vi "Inference(Image)(Batch)(Benchmark).vi"(0 "NNFE PatchCore Paths":T1={"CFG"=path "D:/Ngene/Projects_SVN/DeepLTK/R_and_D/2024_02_01_Patchcore/LabVIEW/NN_Models/PCore_L2L3_Concat_224x224/wrn/wrn_net_cfg_24_08_02__10_26_58.cfg", "BIN"=path "D:/Ngene/Projects_SVN/DeepLTK/R_and_D/2024_02_01_Patchcore/LabVIEW/NN_Models/PCore_L2L3_Concat_224x224/wrn/wrn_weights_24_08_02__10_26_58.bin"}, 1 "NNPC_Setup":T2={"Input_Dims"={"C"=3, "H"=224, "W"=224}, "mBatch"=8, "Device"=enum."GPU", "GPU Id"=0}, 2 "Feature_Scorer_Params":T5={"Nearest_Neighbors"=1, "Calculate Anomaly Map"=TRUE, "Gaussian_Blur"={"Kernel_Size"=33, "Sigma"=4.0}}, 5 "Dataset Folder Path":path=path "D:/DNN/delete/leather/test", 11 "error in":errorcluster) -> (4 "dT_Inf(perImg)(Map=ON)":dbl=0.005463627986157209 format="%#_3ps", 6 "dT_Inf(perImg)(Map=OFF)":dbl=0.00546564111110557 format="%#_3ps", 15 "error out":errorcluster)   [LabVIEW 2024]
uses:
  DeepLTK_Anomaly_Detection_Addon/API/Controls/NNPC_PreProcessing_Options.ctl
  <vilib>/Analysis/NI_AALBase.lvlib
  <vilib>/Analysis/baseanly.llb/Mean (DBL).vi
  DeepLTK_Anomaly_Detection_Addon/API/NNPC_Predict/NNPC_Predict(Batch).vi
  DeepLTK_Anomaly_Detection_Addon/API/Controls/Image_Stats_RGB.ctl
  DeepLTK_Anomaly_Detection_Addon/API/Controls/NNPC_DS_Stats.ctl
  <vilib>/Ngene/Deep Learning Toolkit/Toolkit/NN_Data/API/NN_Dims(C,H,W).ctl
  <vilib>/Ngene/Deep Learning Toolkit/Toolkit/Deep_Learning_Toolkit_by_Ngene.lvlib
  DeepLTK_Anomaly_Detection_Addon/API/Controls/Gaussian_Blur.ctl
  DeepLTK_Anomaly_Detection_Addon/API/Controls/Feature_Scorer_Params.ctl
  DeepLTK_Anomaly_Detection_Addon/API/Controls/NNPC_Setup.ctl
  <vilib>/Ngene/Deep Learning Toolkit/Toolkit/NN_Network/Controls/NN_Device.ctl
  DeepLTK_Anomaly_Detection_Addon/API/Controls/NN_Paths.ctl
panel:
  out "dT_Inf(Map=OFF)":dbl=0.08745025777768912 format="%#_3ps"
  out "dT_ImRead":dbl=0.035323825000887155 format="%#_4ps"
  out "dT_Inf(Map=ON)":dbl=0.08741804777851535 format="%#_3ps"
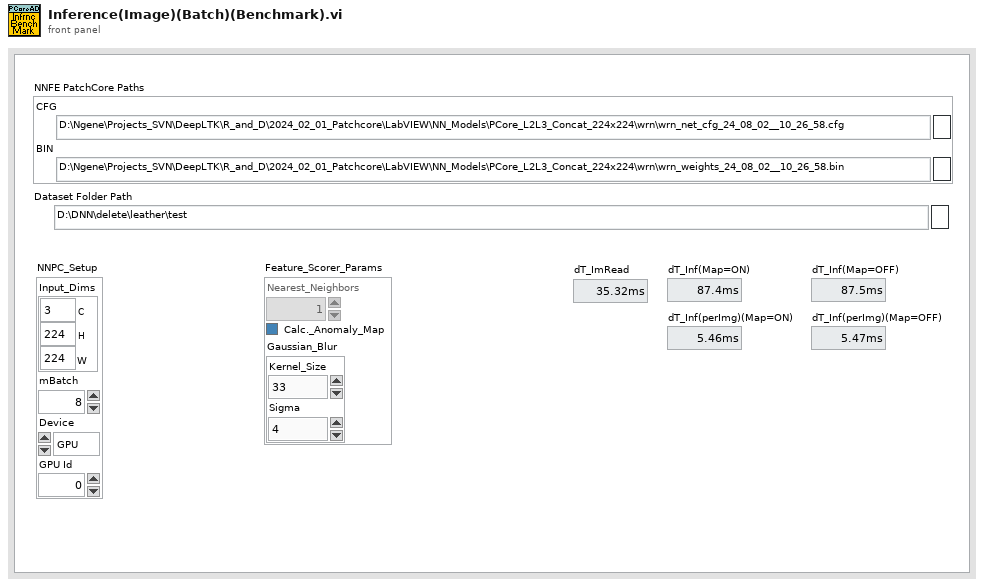
[diagram p1: front panel]
types:
  T1 = typedef "NN_Paths.ctl" = cluster{"CFG":path, "BIN":path}
  T2 = typedef "NNPC_Setup.ctl" = cluster{"Input_Dims":T3, "mBatch":i32, "Device":T4, "GPU Id":i32}
  T3 = typedef "Deep_Learning_Toolkit_by_Ngene.lvlib/NN_Dims(C,H,W).ctl" = cluster{"C":i32, "H":i32, "W":i32}
  T4 = typedef "Deep_Learning_Toolkit_by_Ngene.lvlib/NN_Device.ctl" = enum16{"CPU", "GPU"}
  T5 = typedef "Feature_Scorer_Params.ctl" = cluster{"Nearest_Neighbors":i32, "Calculate Anomaly Map":bool, "Gaussian_Blur":T6}
  T6 = typedef "Gaussian_Blur.ctl" = cluster{"Kernel_Size":i32, "Sigma":sgl}
  T7 = typedef "NNPC_PreProcessing_Options.ctl" = cluster{"DS_Name":string, "Input_Dims":T3, "Center Crop Size":i32, "Interpolation Type":u32, "Dataset_Stats":T8, "Multi-Stage_DownSample?":bool}
  T8 = typedef "NNPC_DS_Stats.ctl" = cluster{"means":T9, "stds":T9}
  T9 = typedef "Image_Stats_RGB.ctl" = cluster{"R":sgl, "G":sgl, "B":sgl}
  T10 = typedef "NNPC_Instance.ctl" = cluster{"NN":T11, "MemBank_Data":T26, "Name":string}
  T11 = typedef "Deep_Learning_Toolkit_by_Ngene.lvlib/NN.ctl" = cluster{"Name":string, "No of Layers":i32, "mBatch":i32, "Layers":T12[], "Dimty":T13, "Dims_In":T3, "Dims_Out":T3, "Working_Dir":path, "Train?":bool, "Train_Params":T14, "LR_Update_Policy":T17, "Session Data":T19, "Ground_truth":T20, "NNg_hdls":T21, "NN_Device":T4, "GPU Id":i32, "Labels":string[], "Receptive Field":T22[], "Loss_Type":T23, "Loss_Cfg_Prms":variant, "NNG_WS":T24}
  T12 = typedef "Deep_Learning_Toolkit_by_Ngene.lvlib/NN_Layer_ref.ctl" = refnum<data-value>
  T13 = typedef "Deep_Learning_Toolkit_by_Ngene.lvlib/NN_In_Out_Dim-ty.ctl" = enum8{"In1D_Out1D", "In3D_Out1D", "In3D_Out3D", "In3D_OutBBox"}
  T14 = typedef "Deep_Learning_Toolkit_by_Ngene.lvlib/NN_Train_Params.ctl" = cluster{"Optimizer":T15, "Beta_1":sgl, "Beta_2":sgl, "Weight Decay(L1)":sgl, "Weight Decay(L2)":sgl, "Data_Sampling":T16}
  T15 = typedef "Deep_Learning_Toolkit_by_Ngene.lvlib/NN_Train_Optimizer.ctl" = enum16{"SGD", "Adam", "Adagrad", "Adadelta", "RMSProp", "Nesterov"}
  T16 = typedef "Deep_Learning_Toolkit_by_Ngene.lvlib/NN_Train_Data_Sampling.ctl" = enum16{"Random", "Sequential"}
  T17 = typedef "Deep_Learning_Toolkit_by_Ngene.lvlib/NN_LR_Policy_Cfg.ctl" = cluster{"Policy_Type":T18, "LR0":dbl, "k":sgl, "WarmUp_Policy":enum16{"Step", "Ramp"}, "WarmUp_Iter":i32, "WarmUp_Ratio":sgl}
  T18 = typedef "Deep_Learning_Toolkit_by_Ngene.lvlib/NN_LR_Policy_Type.ctl" = enum16{"Manual", "Step", "Exp", "1/t"}
  T19 = typedef "Deep_Learning_Toolkit_by_Ngene.lvlib/NN_Train_Session_Data.ctl" = cluster{"Epochs":sgl, "Tot_Iter":i32, "LR":sgl, "LR_iter":i32}
  T20 = typedef "Deep_Learning_Toolkit_by_Ngene.lvlib/NN_Ground_truth.ctl" = cluster{"Y":variant}
  T21 = typedef "Deep_Learning_Toolkit_by_Ngene.lvlib/nng_cuda_handles.ctl" = cluster{"cudnn":u64, "cublas":u64, "stream":u64, "curand":u64}
  T22 = typedef "Deep_Learning_Toolkit_by_Ngene.lvlib/NN_Dims(V,H).ctl" = cluster{"V":i32, "H":i32}
  T23 = typedef "Deep_Learning_Toolkit_by_Ngene.lvlib/NN_Loss_Type.ctl" = enum16{"None", "MSE", "CrossEntropy", "YOLO_v2", "YOLO_v4"}
  T24 = typedef "Deep_Learning_Toolkit_by_Ngene.lvlib/NNG_WS.ctl" = cluster{"NNG_WS_Mem":T25, "Max_WS_Size":i64}
  T25 = typedef "Deep_Learning_Toolkit_by_Ngene.lvlib/NNg_WS_Mem_DVR.ctl" = refnum<data-value>
  T26 = typedef "MemBank_and_Norm_Variants.ctl" = cluster{"MemBank":variant, "MemBank Norm":variant}
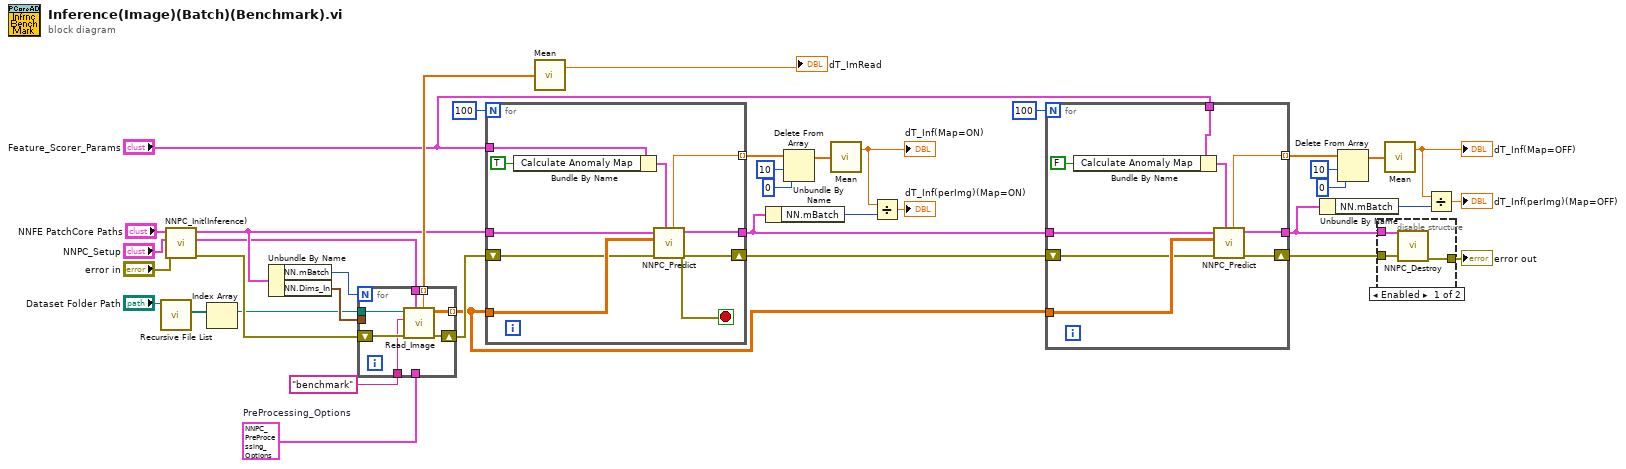
[diagram p0: block diagram]
diagram:
  w37 = T7 {"DS_Name"="", "Input_Dims"={"C"=0, "H"=224, "W"=224}, "Center Crop Size"=-1, "Interpolation Type"=1, "Dataset_Stats"={"means"={"R"=0.5385, "G"=0.5348, "B"=0.551}, "stds"={"R"=0.3673, "G"=0.3673, "B"=0.3505}}, "Multi-Stage_DownSample?"=FALSE}  # PreProcessing_Options
  n1 = call <vilib>:"Recursive File List.vi"("Folder Path"="Dataset Folder Path") -> ("All Files in Dir"=w8:path[])  [unwired: 6 in, 4 out]
  n2 = call "NNPC_Init(Inference).vi"("error in"="error in", "NNPC_Setup"="NNPC_Setup", "NNPC_Paths"="NNFE PatchCore Paths") -> ("error out"=w36:errorcluster, "PreProc_Options"=w2:T7, "NNPC_out"=w5:T10)  [unwired: 4 in, 2 out]
  n3 = Index Array(array=w8) -> (element=w7:path)  [unwired: 1 in]
  n4 = Unbundle By Name(w5) -> ("NN.mBatch"=w32:i32, "NN.Dims_In"=w35:T3)
  n5 = for {
    N: w32 -> [_]
    tunnel: [w46] -> w30 mode=indexing
    tunnel: [w45] -> w14 mode=indexing
    tunnel: w37 -> [_]
    shift-right: [w42] -> w34
    shift-left: w36 -> [w43]
    tunnel: w35 -> [_]
    tunnel: w7 -> [w44]
    tunnel: "benchmark" ("IMAQ Name") -> [w41]
    tunnel: w2 -> [w40]
    n6 = call "Read_Image.vi"("PreProcessing_Options"=w40, "error in"=w43, "IMAQ Name"=w41, "Img Path"=w44) -> ("error out"=w42:errorcluster, "Image Out"=w45:sgl[][][], "dT_Img_Read"=w46:dbl)  [unwired: 4 in, 1 out]
  }
  n7 = for {
    N: 100 -> [_]
    tunnel: w5 -> [w55]
    tunnel: [w54] -> w16
    tunnel: w14 -> [w53]
    tunnel: "Feature_Scorer_Params" -> [w51]
    tunnel: [w48] -> w26 mode=indexing
    shift-right: [w47] -> w15
    shift-left: w34 -> [w52]
    stop <- w47 stop-if-true
    n8 = Bundle By Name(cluster=w51, "Calculate Anomaly Map"=TRUE) -> (w50:T5)
    n9 = call-poly "NNPC_Predict.vi"("Feature_Scorer_Params"=w50, "error in (no error)"=w52, "Image(Batch)"=w53, "NNPC_in"=w55) -> ("error out"=w47:errorcluster, "NNPC_out"=w54:T10, "dT_Predict"=w48:dbl)  [unwired: 3 in, 2 out]
  }
  n10 = call-poly <vilib>:"Mean.vi"("X"=w30) -> ("mean"=→"dT_ImRead":dbl)  [unwired: 1 out]
  n11 = Unbundle By Name(w16) -> ("NN.mBatch"=w29:i32)
  n12 = Delete From Array(array=w26, length=10, index=0) -> (array with subset deleted=w25:dbl[])  [unwired: 1 out]
  n13 = call-poly <vilib>:"Mean.vi"("X"=w25) -> ("mean"=w27:dbl)  [unwired: 1 out]
  "dT_Inf(Map=ON)" <- w27
  n14 = Divide(x=w27, y=w29) -> (x/y=→"dT_Inf(perImg)(Map=ON)":dbl)
  n15 = for {
    N: 100 -> [_]
    tunnel: w16 -> [w64]
    tunnel: [w63] -> w6
    tunnel: w14 -> [w62]
    tunnel: "Feature_Scorer_Params" -> [w60]
    tunnel: [w57] -> w19 mode=indexing
    shift-right: [w56] -> w11
    shift-left: w15 -> [w61]
    n16 = Bundle By Name(cluster=w60, "Calculate Anomaly Map"=FALSE) -> (w59:T5)
    n17 = call-poly "NNPC_Predict.vi"("Feature_Scorer_Params"=w59, "error in (no error)"=w61, "Image(Batch)"=w62, "NNPC_in"=w64) -> ("error out"=w56:errorcluster, "NNPC_out"=w63:T10, "dT_Predict"=w57:dbl)  [unwired: 3 in, 2 out]
  }
  n18 = Unbundle By Name(w6) -> ("NN.mBatch"=w18:i32)
  n19 = Delete From Array(array=w19, length=10, index=0) -> (array with subset deleted=w20:dbl[])  [unwired: 1 out]
  n20 = disable-structure shown="Enabled" {
    disable-tunnel: [w67 w68] -> w39
    disable-tunnel: w6 -> [w66 _]
    disable-tunnel: w11 -> [w65 w68]
    frame Enabled {
      n21 = call "NNPC_Destroy.vi"("error in"=w65, "NNPC_in"=w66) -> ("error out"=w67:errorcluster)  [unwired: 9 in]
    }
    frame Disabled {
    }
  }
  "error out" <- w39
  n22 = call-poly <vilib>:"Mean.vi"("X"=w20) -> ("mean"=w13:dbl)  [unwired: 1 out]
  "dT_Inf(Map=OFF)" <- w13
  n23 = Divide(x=w13, y=w18) -> (x/y=→"dT_Inf(perImg)(Map=OFF)":dbl)
